vi "ep_PQS Calculation.vi"(8 "I phase":dbl[](array[numeric]), 9 "I magnitute":dbl[](array[numeric]), 10 "U phase":dbl[](array[numeric]), 11 "U magnitute":dbl[](array[numeric])) -> (1 "Q":dbl[](array[numeric]), 2 "S":dbl[](array[numeric]), 3 "P":dbl[](array[numeric]))   [LabVIEW 2013, in "NI_EP_Power Measurement.lvlib"]
uses:
  <vilib>/addons/Electrical Power/Power Measurement/NI_EP_Power Measurement.lvlib
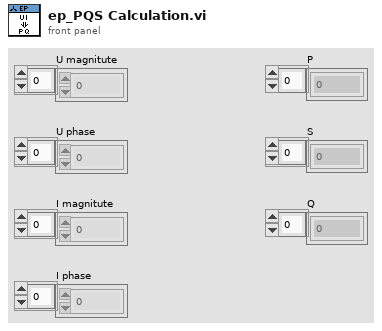
[diagram p1: front panel]
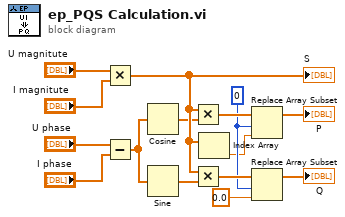
[diagram p0: block diagram]
diagram:
  w4 = 0
  n1 = Multiply(x="U magnitute", y="I magnitute") -> (x*y=w14:dbl[])
  "S" <- w14
  n2 = Subtract(x="U phase", y="I phase") -> (x-y=w15:dbl[])
  n3 = Cosine(x=w15) -> (cos(x)=w12:dbl[])
  n4 = Sine(x=w15) -> (sin(x)=w13:dbl[])
  n5 = Multiply(x=w14, y=w12) -> (x*y=w11:dbl[])
  n6 = Multiply(x=w14, y=w13) -> (x*y=w10:dbl[])
  n7 = Index Array(array=w14) -> (element=w1:dbl)  [unwired: 1 in]
  n8 = Replace Array Subset(array=w11, new element=w1, index=w4) -> (→"P":dbl[])
  n9 = Replace Array Subset(array=w10, new element=0.0, index=w4) -> (→"Q":dbl[])
